vi "集成干预流程.vi"(11 "参数":T1) -> ()   [LabVIEW 2016, in "PLC.lvlib"]
uses:
  PLC.lvlib
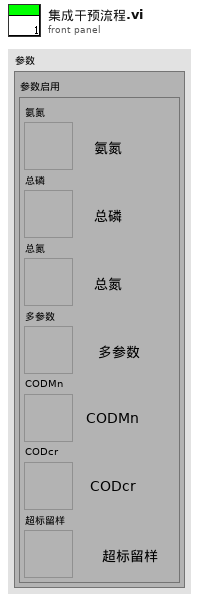
[diagram p1: front panel]
types:
  T1 = cluster{"参数启用":cluster{"氨氮":bool, "总磷":bool, "总氮":bool, "多参数":bool, "CODMn":bool, "CODcr":bool, "超标留样":bool}}
  T2 = enum16{"启动水样测试", "等待测试结束", "获取测试数据", "计算测试结果", "结束"}
  T3 = cluster{"系统时间":timestamp, "工作状态":u16, "测量模式":enum16{"待机", "连续模式", "周期模式", "定点模式", "受控模式", "手动模式"}, "告警代码":u16, "故障代码":u16, "日志代码":u16, "软件版本":u16, "F0":sgl, "F1":sgl, "F2":sgl, "F3":sgl, "T":sgl, "H":sgl, "id":u16, "flowid":u16, "量程":u16, "总磷控温温度1":sgl, "营养盐控温温度2":sgl, "ADC":sgl}
  T4 = cluster{"系统时间":timestamp, "工作状态":u16, "测量模式":enum16{"待机", "连续模式", "周期模式", "定点模式", "受控模式", "手动模式"}, "告警代码":u16, "故障代码":u16, "日志代码":u16, "软件版本":u16, "F0":sgl, "F1":sgl, "F2":sgl, "F3":sgl, "T":sgl, "H":sgl, "id":u16, "flowid":u16, "量程":u16, "总磷控温温度1":sgl, "营养盐控温温度2":sgl, "ADC":sgl}[]
  T5 = cluster{"时间标识":timestamp, "参数":string, "数据类型":string, "集成干预测试浓度值":dbl, "集成干预前测试时间":timestamp, "集成干预前测试浓度值":dbl}
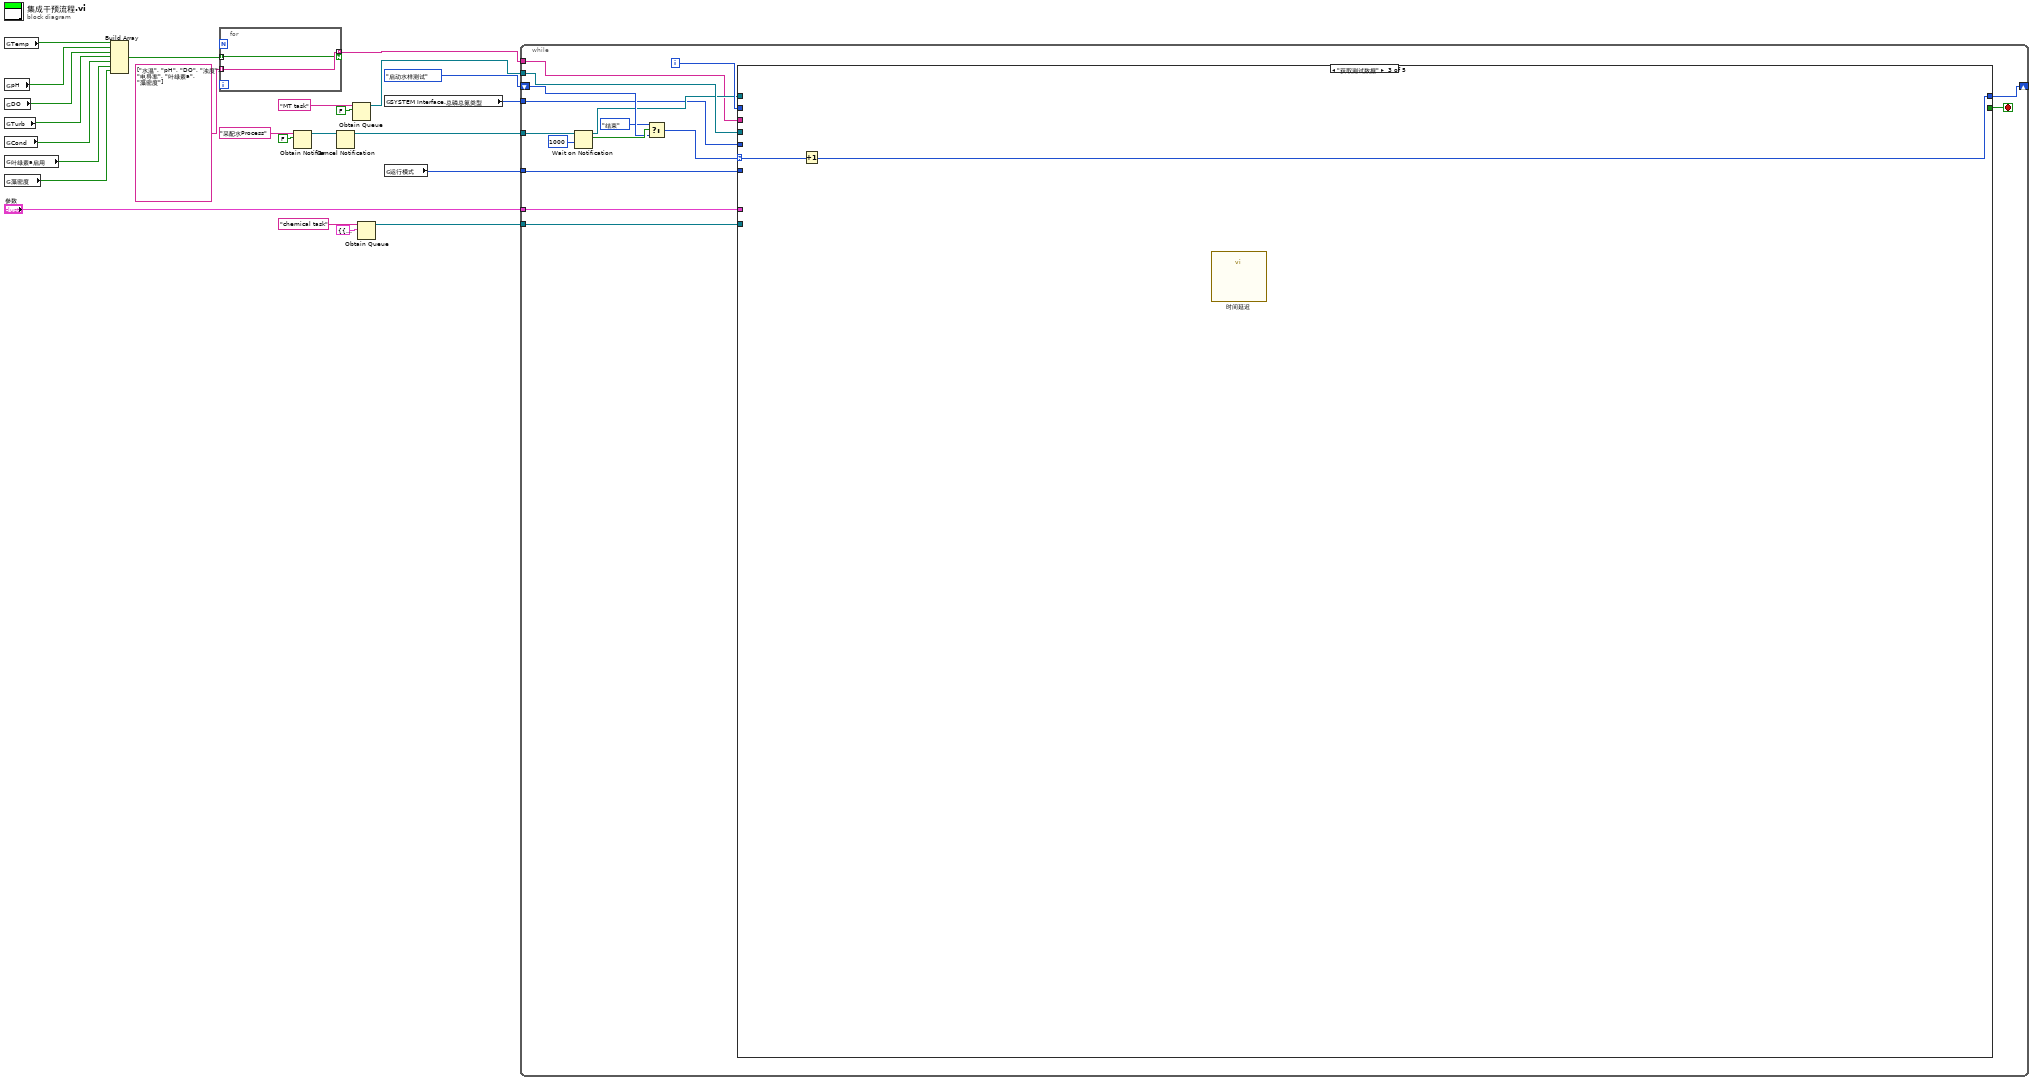
[diagram p0: block diagram]
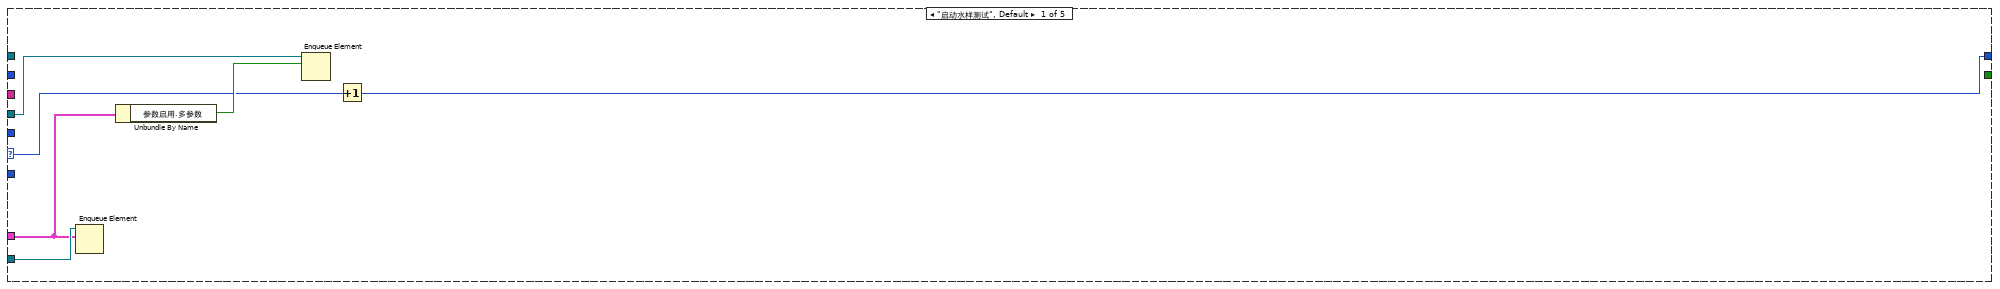
[diagram p2: hidden frame]
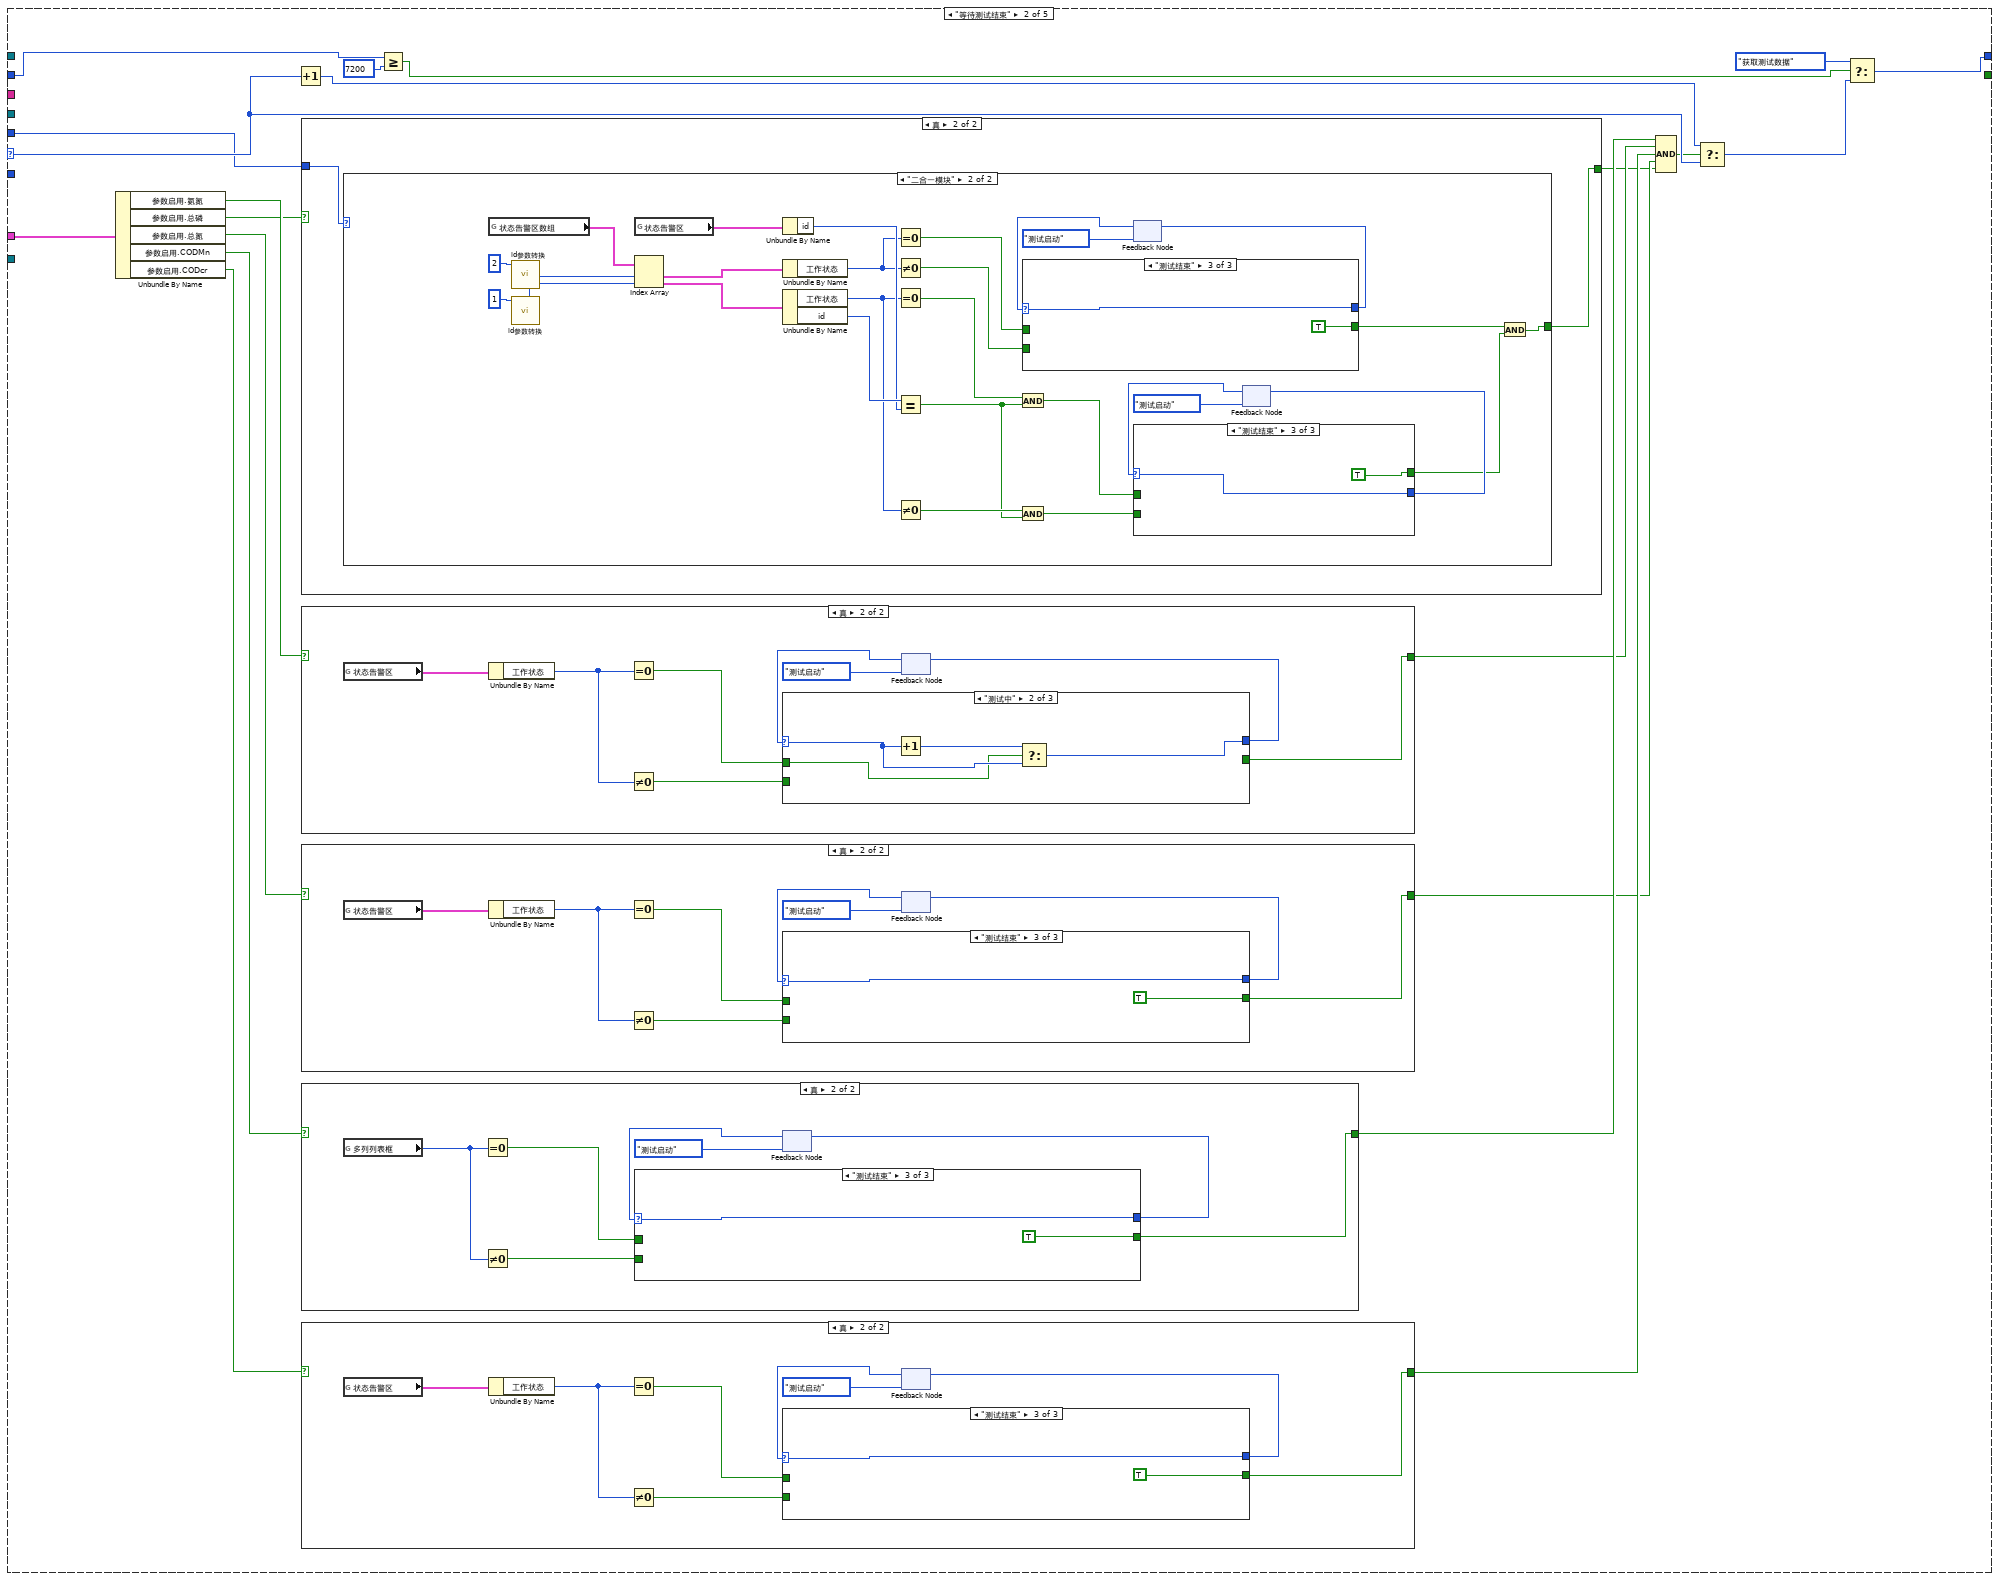
[diagram p3: hidden frame]
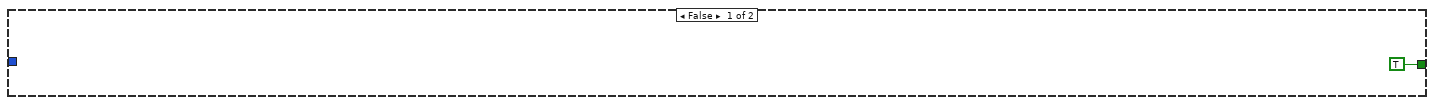
[diagram p4: hidden frame]
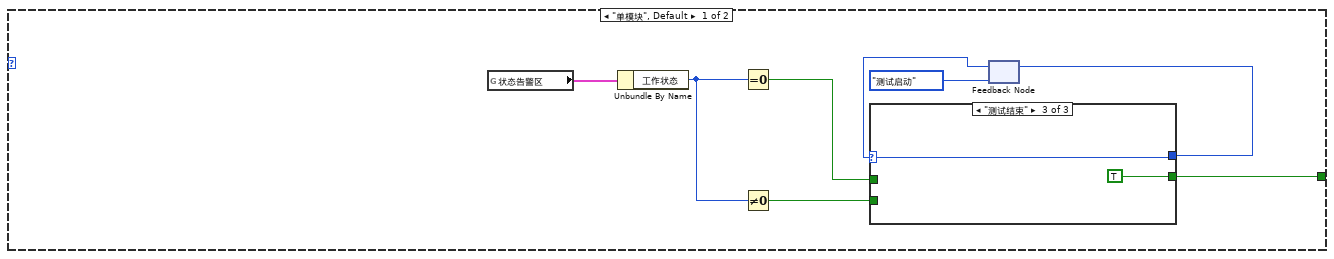
[diagram p5: hidden frame]
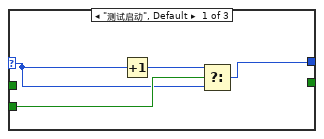
[diagram p6: hidden frame]
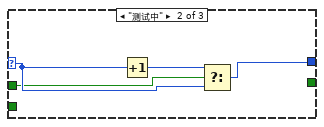
[diagram p7: hidden frame]
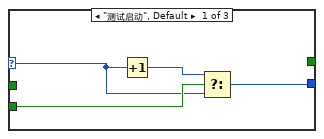
[diagram p8: hidden frame]
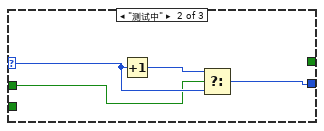
[diagram p9: hidden frame]
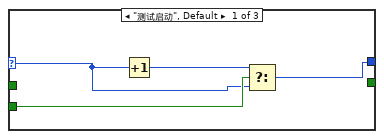
[diagram p10: hidden frame]
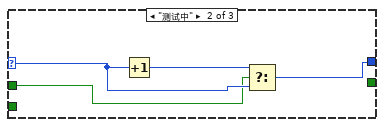
[diagram p11: hidden frame]
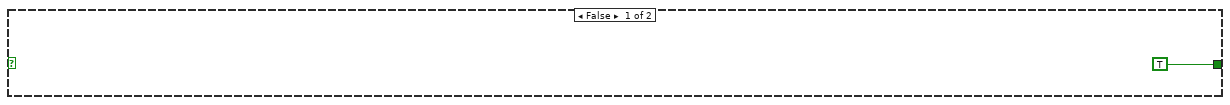
[diagram p12: hidden frame]
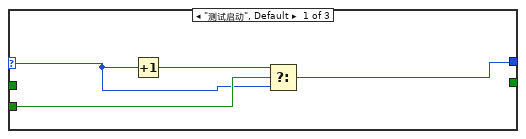
[diagram p13: hidden frame]
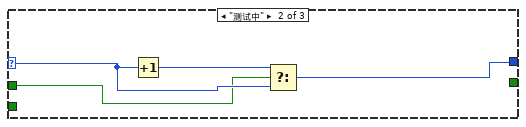
[diagram p14: hidden frame]
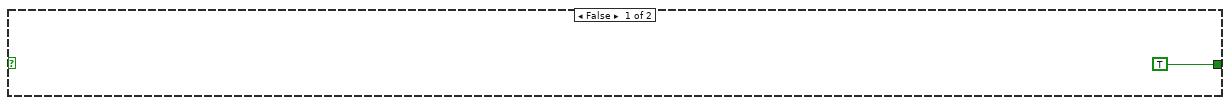
[diagram p15: hidden frame]
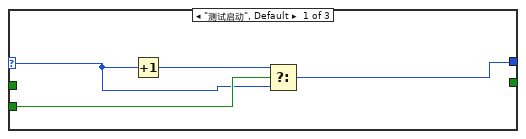
[diagram p16: hidden frame]
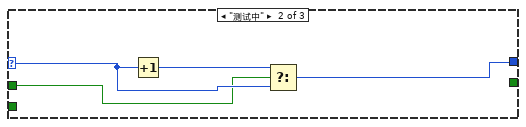
[diagram p17: hidden frame]
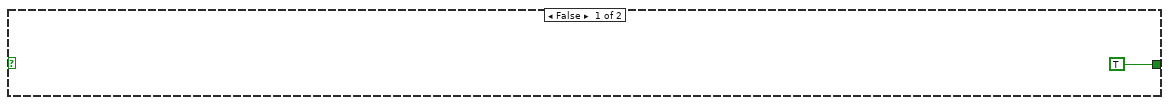
[diagram p18: hidden frame]
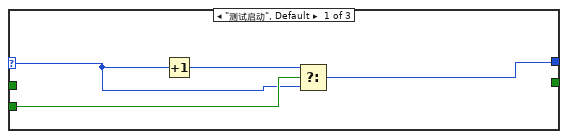
[diagram p19: hidden frame]
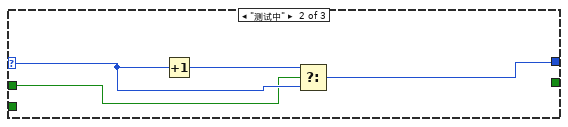
[diagram p20: hidden frame]
diagram:
  n1 = global read "断电保存变量.vi" "Temp"() -> (w2:bool)
  n2 = global read "断电保存变量.vi" "pH"() -> (w3:bool)
  n3 = global read "断电保存变量.vi" "DO"() -> (w8:bool)
  n4 = global read "断电保存变量.vi" "Turb"() -> (w4:bool)
  n5 = global read "断电保存变量.vi" "Cond"() -> (w5:bool)
  n6 = global read "断电保存变量.vi" "叶绿素a启用"() -> (w6:bool)
  n7 = global read "断电保存变量.vi" "藻密度"() -> (w7:bool)
  n8 = Build Array(w2, w3, w8, w4, w5, w6, w7) -> (w9:bool[])
  n9 = for {
    tunnel: w9 -> [w25] mode=indexing
    tunnel: string[] ["水温", "pH", "DO", "浊度", "电导率", "叶绿素a", "藻密度"] -> [w26] mode=indexing
    tunnel: [w26] -> w1 mode=indexing if=w25
  }
  n10 = Obtain Notifier(name (unnamed)="采配水Process" ("名称（未命名）"), notification data type=FALSE) -> (notifier out=w14:refnum<notifier>)  [unwired: 2 in, 2 out]
  n11 = Cancel Notification(0:w14) -> (8:w13:refnum<notifier>)  [unwired: 1 in, 2 out]
  n12 = Obtain Queue(name (unnamed)="MT task" ("名称（未命名）"), element data type=FALSE) -> (queue out=w18:refnum<queue>)  [unwired: 3 in, 2 out]
  n13 = Obtain Queue(name (unnamed)="chemical task" ("名称（未命名）"), element data type=T1 {"参数启用"={"氨氮"=FALSE, "总磷"=FALSE, "总氮"=FALSE, "多参数"=FALSE, "CODMn"=FALSE, "CODcr"=FALSE, "超标留样"=FALSE}} ("参数")) -> (queue out=w19:refnum<queue>)  [unwired: 3 in, 2 out]
  n14 = global read "系统设置全局变量.vi" "SYSTEM Interface.总磷总氮类型"() -> (w11:enum16{"单模块", "二合一模块"})
  n15 = global read "系统设置全局变量.vi" "运行模式"() -> (w12:enum16{"维护模式", "常规模式", "应急模式", "质控模式"})
  n16 = while {
    tunnel: "参数" -> [w41]
    tunnel: w19 -> [w42]
    tunnel: w18 -> [w40]
    shift-right: [w39] -> _
    shift-left: T2."启动水样测试" ("枚举") -> [w33]
    tunnel: w13 -> [w36]
    tunnel: w12 -> [w29]
    tunnel: w11 -> [w28]
    tunnel: w1 -> [w27]
    i -> [w37]
    stop <- w38 stop-if-true
    n17 = Wait on Notification(notifier=w36, timeout in ms (-1)=1000 ("超时毫秒(-1)")) -> (notifier out=w30:refnum<notifier>, notification=w34:bool)  [unwired: 2 in, 2 out]
    n18 = Select(t=T2."结束", s=w34, f=w33) -> (s? t:f=w31:T2)
    n19 = case shown="\"获取测试数据\"" w31 {
      selector: w31 -> [w44 w67 w215 w229 w261]
      tunnel: w42 -> [w48 _ _ _ w260]
      tunnel: w41 -> [w47 w66 _ w227 _]
      tunnel: w40 -> [w46 _ _ _ w259]
      tunnel: [w43 w50 w214 w228 w261] -> w39
      tunnel: [_ _ _ _ TRUE] -> w38
      tunnel: w37 -> [_ w69 _ _ _]
      tunnel: w30 -> [_ _ _ _ w258]
      tunnel: w29 -> [_ _ _ w226 _]
      tunnel: w28 -> [_ w60 _ w217 _]
      tunnel: w27 -> [_ _ _ w216 _]
      frame "启动水样测试", Default {
        n20 = Enqueue Element(queue=w48, element=w47) -> ()  [unwired: 2 in, 3 out]
        n21 = Unbundle By Name(w47) -> ("参数启用.多参数"=w45:bool)
        n22 = Enqueue Element(queue=w46, element=w45) -> ()  [unwired: 2 in, 3 out]
        n23 = Increment(x=w44) -> (x+1=w43:T2)
      }
      frame "等待测试结束" {
        n24 = Unbundle By Name(w66) -> ("参数启用.氨氮"=w65:bool, "参数启用.总磷"=w61:bool, "参数启用.总氮"=w62:bool, "参数启用.CODMn"=w64:bool, "参数启用.CODcr"=w63:bool)
        n25 = Increment(x=w67) -> (x+1=w53:T2)
        n26 = case shown="真" w61 {
          tunnel: [TRUE w72] -> w55
          tunnel: w60 -> [_ w71]
          frame False {
          }
          frame True {
            n27 = case shown="\"二合一模块\"" w71 {
              tunnel: [w73 w108] -> w72
              frame "单模块", Default {
                n28 = global read "VAR总磷总氮全局变量.vi" "状态告警区"() -> (w80:T3)
                n29 = Unbundle By Name(w80) -> ("工作状态"=w75:u16)
                n30 = Equal To 0?(x=w75) -> (x = 0?=w74:bool)
                n31 = Not Equal To 0?(x=w75) -> (x != 0?=w76:bool)
                n32 = feedback #1(enum16{"测试启动", "测试中", "测试结束"}."测试启动" ("枚举")) -> (w78:enum16{"测试启动", "测试中", "测试结束"})
                n33 = case shown="\"测试结束\"" w78 {
                  selector: w78 -> [w82 w87 w90]
                  tunnel: w76 -> [w84 _ _]
                  tunnel: [w81 w86 w90] -> w79
                  tunnel: w74 -> [_ w85 _]
                  tunnel: [_ _ TRUE] -> w73
                  frame "测试启动", Default {
                    n34 = Increment(x=w82) -> (x+1=w83:enum16{"测试启动", "测试中", "测试结束"})
                    n35 = Select(t=w83, s=w84, f=w82) -> (s? t:f=w81:enum16{"测试启动", "测试中", "测试结束"})
                  }
                  frame "测试中" {
                    n36 = Increment(x=w87) -> (x+1=w88:enum16{"测试启动", "测试中", "测试结束"})
                    n37 = Select(t=w88, s=w85, f=w87) -> (s? t:f=w86:enum16{"测试启动", "测试中", "测试结束"})
                  }
                  frame "测试结束" {
                  }
                }
                n38 = feedback-in #1(w79) -> ()
              }
              frame "二合一模块" {
                n39 = global read "VAR总磷总氮全局变量.vi" "状态告警区数组"() -> (w115:T4)
                n40 = call "id参数转换.vi"("id"=u16 2) -> ("数组资源索引"=w116:i32)  [unwired: 9 in, 1 out]
                n41 = call "id参数转换.vi"("id"=u16 1) -> ("数组资源索引"=w118:i32)  [unwired: 9 in, 1 out]
                n42 = global read "VAR总磷总氮全局变量.vi" "状态告警区"() -> (w111:T3)
                n43 = Index Array(array=w115, index #1=w116, index #2=w118) -> (element #1=w113:T3, element #2=w112:T3)
                n44 = Unbundle By Name(w111) -> ("id"=w109:u16)
                n45 = Unbundle By Name(w113) -> ("工作状态"=w99:u16)
                n46 = Unbundle By Name(w112) -> ("工作状态"=w94:u16, "id"=w110:u16)
                n47 = Equal To 0?(x=w99) -> (x = 0?=w100:bool)
                n48 = Not Equal To 0?(x=w99) -> (x != 0?=w98:bool)
                n49 = Equal To 0?(x=w94) -> (x = 0?=w107:bool)
                n50 = Equal?(x=w110, y=w109) -> (x = y?=w93:bool)
                n51 = Not Equal To 0?(x=w94) -> (x != 0?=w95:bool)
                n52 = And(x=w107, y=w93) -> (x .and. y?=w96:bool)
                n53 = And(x=w95, y=w93) -> (x .and. y?=w92:bool)
                n54 = feedback #2(enum16{"测试启动", "测试中", "测试结束"}."测试启动" ("枚举")) -> (w105:enum16{"测试启动", "测试中", "测试结束"})
                n55 = case shown="\"测试结束\"" w105 {
                  selector: w105 -> [w130 w135 w138]
                  tunnel: w98 -> [w132 _ _]
                  tunnel: [w129 w134 w138] -> w106
                  tunnel: w100 -> [_ w133 _]
                  tunnel: [_ _ TRUE] -> w97
                  frame "测试启动", Default {
                    n56 = Increment(x=w130) -> (x+1=w131:enum16{"测试启动", "测试中", "测试结束"})
                    n57 = Select(t=w131, s=w132, f=w130) -> (s? t:f=w129:enum16{"测试启动", "测试中", "测试结束"})
                  }
                  frame "测试中" {
                    n58 = Increment(x=w135) -> (x+1=w136:enum16{"测试启动", "测试中", "测试结束"})
                    n59 = Select(t=w136, s=w133, f=w135) -> (s? t:f=w134:enum16{"测试启动", "测试中", "测试结束"})
                  }
                  frame "测试结束" {
                  }
                }
                n60 = feedback-in #2(w106) -> ()
                n61 = feedback #3(enum16{"测试启动", "测试中", "测试结束"}."测试启动" ("枚举")) -> (w102:enum16{"测试启动", "测试中", "测试结束"})
                n62 = case shown="\"测试结束\"" w102 {
                  selector: w102 -> [w120 w125 w128]
                  tunnel: w92 -> [w122 _ _]
                  tunnel: [w119 w124 w128] -> w101
                  tunnel: w96 -> [_ w123 _]
                  tunnel: [_ _ TRUE] -> w91
                  frame "测试启动", Default {
                    n63 = Increment(x=w120) -> (x+1=w121:enum16{"测试启动", "测试中", "测试结束"})
                    n64 = Select(t=w121, s=w122, f=w120) -> (s? t:f=w119:enum16{"测试启动", "测试中", "测试结束"})
                  }
                  frame "测试中" {
                    n65 = Increment(x=w125) -> (x+1=w126:enum16{"测试启动", "测试中", "测试结束"})
                    n66 = Select(t=w126, s=w123, f=w125) -> (s? t:f=w124:enum16{"测试启动", "测试中", "测试结束"})
                  }
                  frame "测试结束" {
                  }
                }
                n67 = feedback-in #3(w101) -> ()
                n68 = And(x=w97, y=w91) -> (x .and. y?=w108:bool)
              }
            }
          }
        }
        n69 = case shown="真" w65 {
          tunnel: [TRUE w196] -> w58
          frame False {
          }
          frame True {
            n70 = global read "VAR总磷总氮全局变量.vi" "状态告警区"() -> (w203:T3)
            n71 = Unbundle By Name(w203) -> ("工作状态"=w199:u16)
            n72 = Equal To 0?(x=w199) -> (x = 0?=w197:bool)
            n73 = Not Equal To 0?(x=w199) -> (x != 0?=w198:bool)
            n74 = feedback #4(enum16{"测试启动", "测试中", "测试结束"}."测试启动" ("枚举")) -> (w201:enum16{"测试启动", "测试中", "测试结束"})
            n75 = case shown="\"测试中\"" w201 {
              selector: w201 -> [w205 w210 w213]
              tunnel: w198 -> [w207 _ _]
              tunnel: [w204 w209 w213] -> w202
              tunnel: w197 -> [_ w208 _]
              tunnel: [_ _ TRUE] -> w196
              frame "测试启动", Default {
                n76 = Increment(x=w205) -> (x+1=w206:enum16{"测试启动", "测试中", "测试结束"})
                n77 = Select(t=w206, s=w207, f=w205) -> (s? t:f=w204:enum16{"测试启动", "测试中", "测试结束"})
              }
              frame "测试中" {
                n78 = Increment(x=w210) -> (x+1=w211:enum16{"测试启动", "测试中", "测试结束"})
                n79 = Select(t=w211, s=w208, f=w210) -> (s? t:f=w209:enum16{"测试启动", "测试中", "测试结束"})
              }
              frame "测试结束" {
              }
            }
            n80 = feedback-in #4(w202) -> ()
          }
        }
        n81 = case shown="真" w62 {
          tunnel: [TRUE w143] -> w56
          frame False {
          }
          frame True {
            n82 = global read "VAR总磷总氮全局变量.vi" "状态告警区"() -> (w147:T3)
            n83 = Unbundle By Name(w147) -> ("工作状态"=w141:u16)
            n84 = Equal To 0?(x=w141) -> (x = 0?=w142:bool)
            n85 = Not Equal To 0?(x=w141) -> (x != 0?=w140:bool)
            n86 = feedback #5(enum16{"测试启动", "测试中", "测试结束"}."测试启动" ("枚举")) -> (w145:enum16{"测试启动", "测试中", "测试结束"})
            n87 = case shown="\"测试结束\"" w145 {
              selector: w145 -> [w149 w154 w157]
              tunnel: w140 -> [w151 _ _]
              tunnel: [w148 w153 w157] -> w146
              tunnel: w142 -> [_ w152 _]
              tunnel: [_ _ TRUE] -> w143
              frame "测试启动", Default {
                n88 = Increment(x=w149) -> (x+1=w150:enum16{"测试启动", "测试中", "测试结束"})
                n89 = Select(t=w150, s=w151, f=w149) -> (s? t:f=w148:enum16{"测试启动", "测试中", "测试结束"})
              }
              frame "测试中" {
                n90 = Increment(x=w154) -> (x+1=w155:enum16{"测试启动", "测试中", "测试结束"})
                n91 = Select(t=w155, s=w152, f=w154) -> (s? t:f=w153:enum16{"测试启动", "测试中", "测试结束"})
              }
              frame "测试结束" {
              }
            }
            n92 = feedback-in #5(w146) -> ()
          }
        }
        n93 = case shown="真" w64 {
          tunnel: [TRUE w180] -> w59
          frame False {
          }
          frame True {
            n94 = global read "运行时序全局变量.vi" "多列列表框"() -> (w179:i32)
            n95 = Equal To 0?(x=w179) -> (x = 0?=w181:bool)
            n96 = Not Equal To 0?(x=w179) -> (x != 0?=w178:bool)
            n97 = feedback #6(enum16{"测试启动", "测试中", "测试结束"}."测试启动" ("枚举")) -> (w183:enum16{"测试启动", "测试中", "测试结束"})
            n98 = case shown="\"测试结束\"" w183 {
              selector: w183 -> [w186 w191 w194]
              tunnel: w178 -> [w188 _ _]
              tunnel: [w185 w190 w194] -> w184
              tunnel: w181 -> [_ w189 _]
              tunnel: [_ _ TRUE] -> w180
              frame "测试启动", Default {
                n99 = Increment(x=w186) -> (x+1=w187:enum16{"测试启动", "测试中", "测试结束"})
                n100 = Select(t=w187, s=w188, f=w186) -> (s? t:f=w185:enum16{"测试启动", "测试中", "测试结束"})
              }
              frame "测试中" {
                n101 = Increment(x=w191) -> (x+1=w192:enum16{"测试启动", "测试中", "测试结束"})
                n102 = Select(t=w192, s=w189, f=w191) -> (s? t:f=w190:enum16{"测试启动", "测试中", "测试结束"})
              }
              frame "测试结束" {
              }
            }
            n103 = feedback-in #6(w184) -> ()
          }
        }
        n104 = case shown="真" w63 {
          tunnel: [TRUE w162] -> w57
          frame False {
          }
          frame True {
            n105 = global read "VAR总磷总氮全局变量.vi" "状态告警区"() -> (w166:T3)
            n106 = Unbundle By Name(w166) -> ("工作状态"=w160:u16)
            n107 = Equal To 0?(x=w160) -> (x = 0?=w161:bool)
            n108 = Not Equal To 0?(x=w160) -> (x != 0?=w159:bool)
            n109 = feedback #7(enum16{"测试启动", "测试中", "测试结束"}."测试启动" ("枚举")) -> (w164:enum16{"测试启动", "测试中", "测试结束"})
            n110 = case shown="\"测试结束\"" w164 {
              selector: w164 -> [w168 w173 w176]
              tunnel: w159 -> [w170 _ _]
              tunnel: [w167 w172 w176] -> w165
              tunnel: w161 -> [_ w171 _]
              tunnel: [_ _ TRUE] -> w162
              frame "测试启动", Default {
                n111 = Increment(x=w168) -> (x+1=w169:enum16{"测试启动", "测试中", "测试结束"})
                n112 = Select(t=w169, s=w170, f=w168) -> (s? t:f=w167:enum16{"测试启动", "测试中", "测试结束"})
              }
              frame "测试中" {
                n113 = Increment(x=w173) -> (x+1=w174:enum16{"测试启动", "测试中", "测试结束"})
                n114 = Select(t=w174, s=w171, f=w173) -> (s? t:f=w172:enum16{"测试启动", "测试中", "测试结束"})
              }
              frame "测试结束" {
              }
            }
            n115 = feedback-in #7(w165) -> ()
          }
        }
        n116 = Greater Or Equal?(x=w69, y=7200) -> (x >= y?=w52:bool)
        n117 = Compound Arithmetic op=AND ("复合运算")(w59, w58, w57, w56, w55) -> (w54:bool)
        n118 = Select(t=w53, s=w54, f=w67) -> (s? t:f=w51:T2)
        n119 = Select(t=T2."获取测试数据", s=w52, f=w51) -> (s? t:f=w50:T2)
      }
      frame "获取测试数据" {
        n120 = Increment(x=w215) -> (x+1=w214:T2)
        n121 = call "时间延迟"() -> ()  [unwired: 11 in, 1 out]
      }
      frame "计算测试结果" {
        n122 = Unbundle By Name(w227) -> ("参数启用.氨氮"=w225:bool, "参数启用.总磷"=w224:bool, "参数启用.总氮"=w223:bool, "参数启用.多参数"=w222:bool, "参数启用.CODMn"=w221:bool, "参数启用.CODcr"=w220:bool)
        n123 = Build Array(w225, w224, w223, w222, w221, w220) -> (w219:bool[])
        n124 = Increment(x=w229) -> (x+1=w228:T2)
        n125 = for {
          tunnel: w226 -> [w235]
          tunnel: w219 -> [w230] mode=indexing
          tunnel: string[] ["氨氮", "总磷", "总氮", "多参数", "CODMn", "CODCr"] -> [w233] mode=indexing
          tunnel: [w234] -> _ mode=indexing
          tunnel: w217 -> [w232]
          tunnel: w216 -> [w231]
          n126 = case shown="真" w230 {
            tunnel: w235 -> [_ w241]
            tunnel: [_ w240] -> w234
            tunnel: w233 -> [_ w239]
            tunnel: w232 -> [_ w237]
            tunnel: w231 -> [_ w236]
            frame False {
            }
            frame True {
              n127 = case shown="默认" w239 {
                selector: w239 -> [w249 _ _]
                tunnel: [w248 w250 w257] -> w238
                tunnel: w237 -> [_ w251 _]
                tunnel: w236 -> [_ _ w257]
                frame Default {
                  n128 = Build Array(w249) -> (w248:string[])
                }
                frame "总磷" {
                  n129 = case shown="\"二合一模块\"" w251 {
                    tunnel: [w252 w254] -> w250
                    frame "单模块", Default {
                      n130 = Build Array("总磷") -> (w252:string[])
                    }
                    frame "二合一模块" {
                      n131 = Build Array("总氮", "总磷") -> (w254:string[])
                    }
                  }
                }
                frame "多参数" {
                }
              }
              n132 = for {
                tunnel: w241 -> [w247]
                tunnel: [w246] -> w240
                tunnel: w238 -> [w243] mode=indexing
                n133 = call "获取最近两组水样测试数据.vi"("运行模式"=w247, "table"=w243) -> ("error out"=w245:errorcluster, "存储变量"=w244:T5)  [unwired: 8 in]
                n134 = call "集成干预测试数据存储.vi"("error in (no error)"=w245, "存储变量"=w244) -> ("error out"=w246:errorcluster)  [unwired: 9 in]
                n135 = Wait (ms)(milliseconds to wait=u32 1000 ("等待时间（毫秒）")) -> ()  [unwired: 1 out]
              }
            }
          }
        }
      }
      frame "结束" {
        n136 = Release Notifier(notifier=w258) -> ()  [unwired: 2 in, 3 out]
        n137 = Release Queue(queue=w259) -> ()  [unwired: 2 in, 3 out]
        n138 = Release Queue(queue=w260) -> ()  [unwired: 2 in, 3 out]
      }
    }
  }
